vi "create_data_header_units.vi"() -> (8 "header units":string)   [LabVIEW 2016]
uses:
  Instrument_Setup.vi
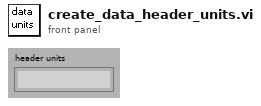
[diagram p1: front panel]
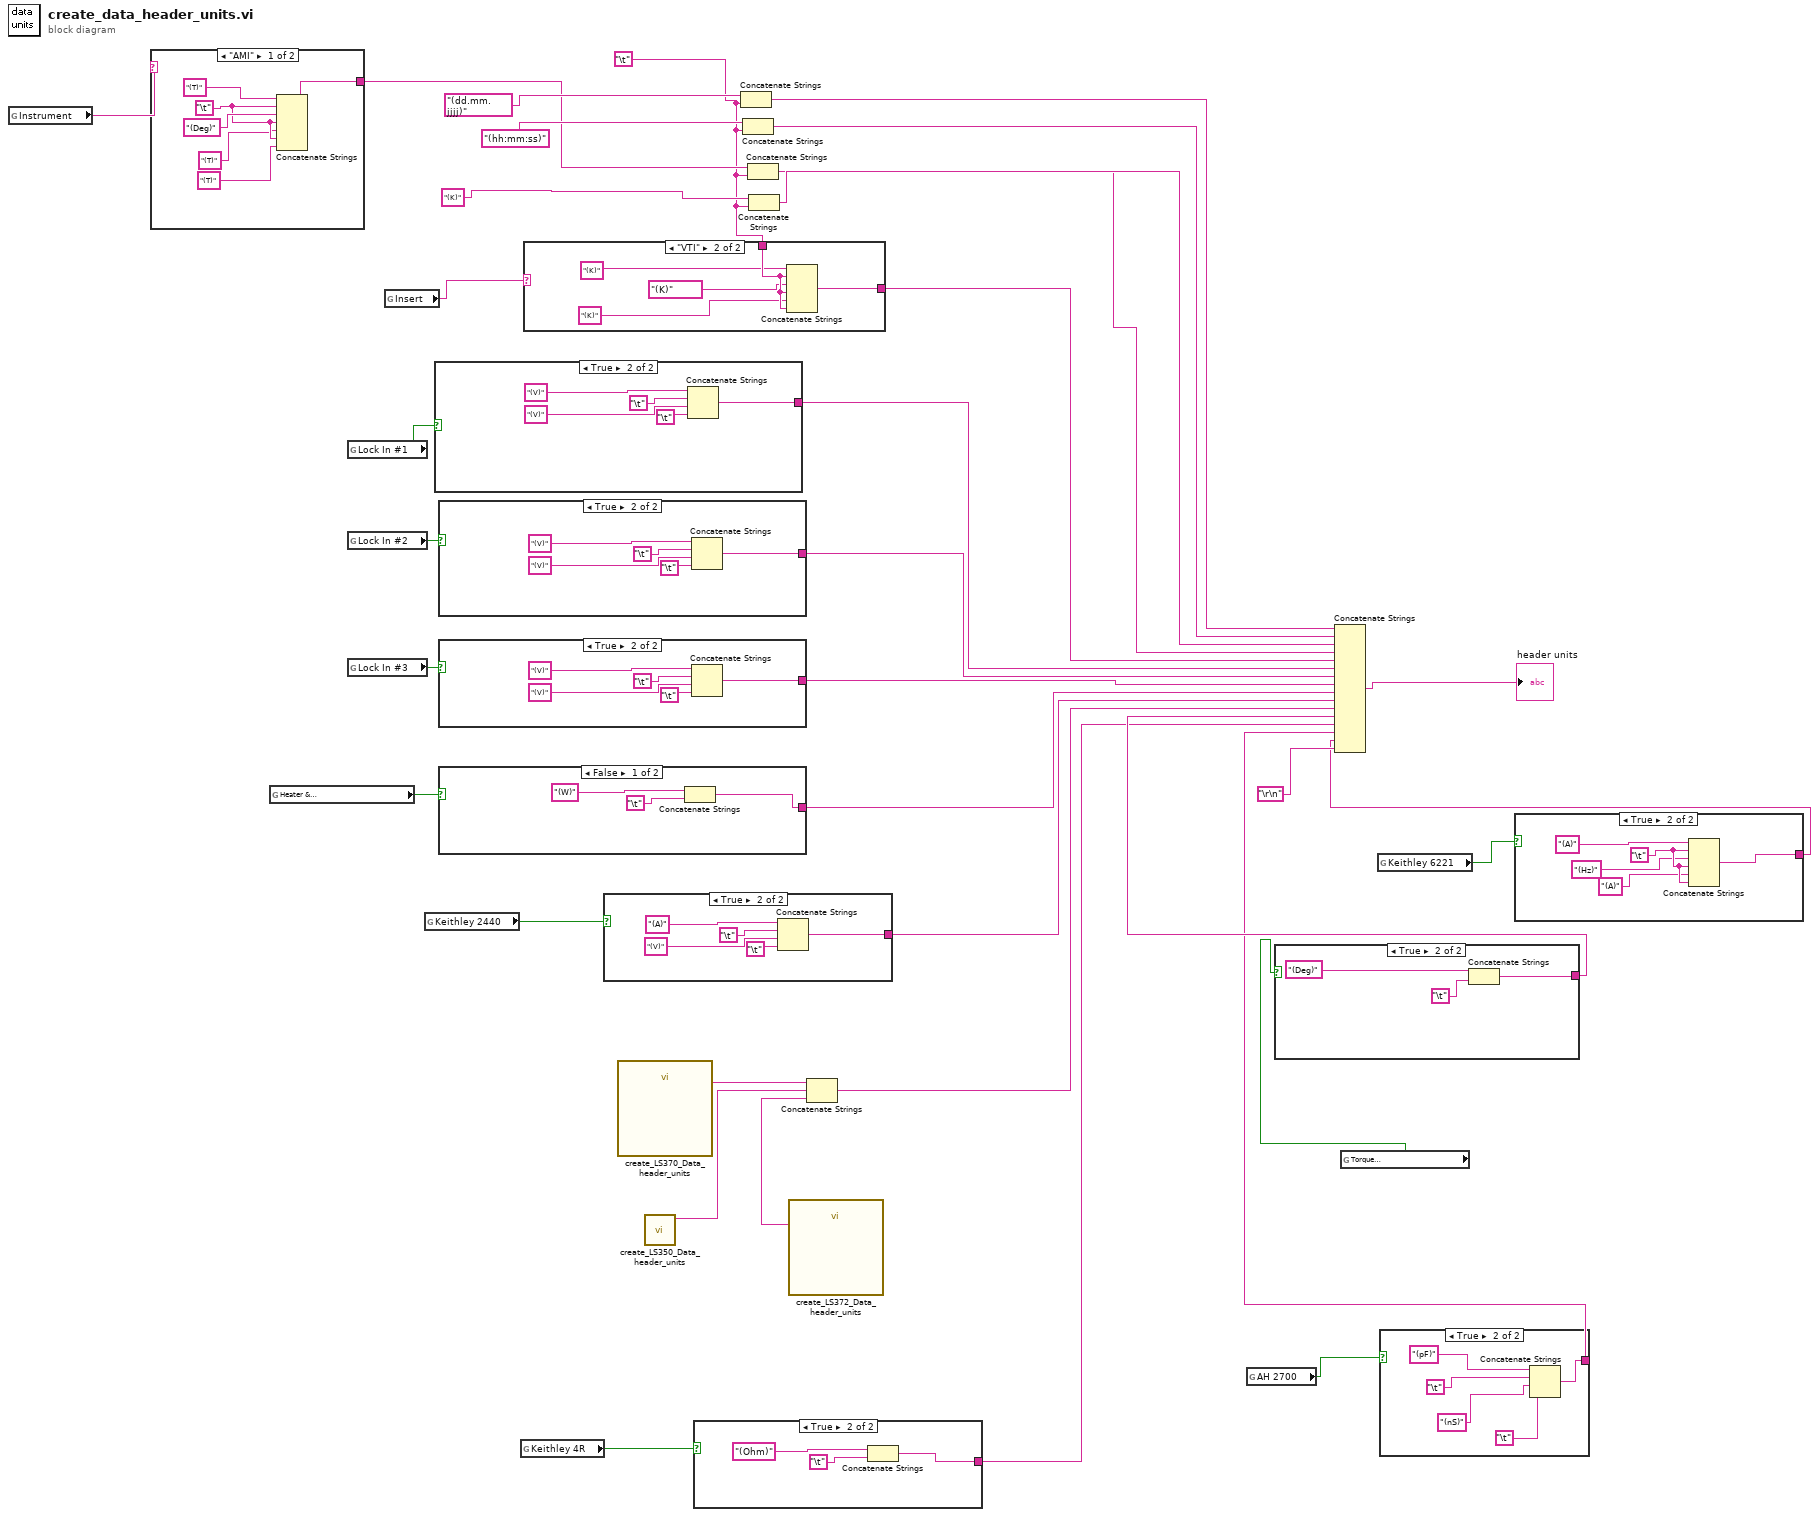
[diagram p0: block diagram]
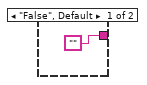
[diagram p2: hidden frame]
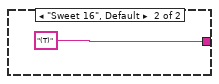
[diagram p3: hidden frame]
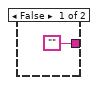
[diagram p4: hidden frame]
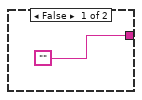
[diagram p5: hidden frame]
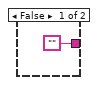
[diagram p6: hidden frame]
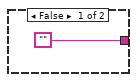
[diagram p7: hidden frame]
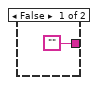
[diagram p8: hidden frame]
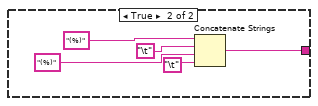
[diagram p9: hidden frame]
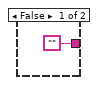
[diagram p10: hidden frame]
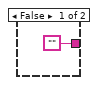
[diagram p11: hidden frame]
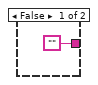
[diagram p12: hidden frame]
diagram:
  w2 = "\t"
  n1 = global read "Instrument_Setup.vi" "Instrument"() -> (w6:string)
  n2 = case shown="\"AMI\"" w6 {
    tunnel: [w40 "(T)"] -> w20
    frame "AMI" {
      w39 = "\t"
      n3 = Concatenate Strings("(T)", w39, "(Deg)", w39, "(T)", w39, "(T)") -> (w40:string)
    }
    frame "Sweet 16", Default {
    }
  }
  n4 = global read "Instrument_Setup.vi" "Heater &\nNeedle Valve"() -> (w33:bool)
  n5 = global read "Instrument_Setup.vi" "Lock In #1"() -> (w36:bool)
  n6 = global read "Instrument_Setup.vi" "Lock In #2"() -> (w35:bool)
  n7 = global read "Instrument_Setup.vi" "Lock In #3"() -> (w34:bool)
  n8 = global read "Instrument_Setup.vi" "Insert"() -> (w3:string)
  n9 = global read "Instrument_Setup.vi" "Keithley 2440"() -> (w32:bool)
  n10 = case shown="True" w36 {
    tunnel: ["" w49] -> w31
    frame False {
    }
    frame True {
      n11 = Concatenate Strings("(V)", "\t", "(V)", "\t") -> (w49:string)
    }
  }
  n12 = case shown="True" w35 {
    tunnel: ["" w51] -> w30
    frame False {
    }
    frame True {
      n13 = Concatenate Strings("(V)", "\t", "(V)", "\t") -> (w51:string)
    }
  }
  n14 = case shown="True" w34 {
    tunnel: ["" w57] -> w29
    frame False {
    }
    frame True {
      n15 = Concatenate Strings("(V)", "\t", "(V)", "\t") -> (w57:string)
    }
  }
  n16 = case shown="False" w33 {
    tunnel: [w62 w69] -> w28
    frame False {
      n17 = Concatenate Strings("(W)", "\t") -> (w62:string)
    }
    frame True {
      n18 = Concatenate Strings("(%)", "\t", "(%)", "\t") -> (w69:string)
    }
  }
  n19 = global read "Instrument_Setup.vi" "Keithley 4R"() -> (w24:bool)
  n20 = case shown="\"VTI\"" w3 {
    tunnel: w2 -> [_ w75]
    tunnel: ["" w74] -> w1
    frame "False", Default {
    }
    frame "VTI" {
      n21 = Concatenate Strings("(K)", w75, "(K)", w75, "(K)", w75) -> (w74:string)
    }
  }
  n22 = case shown="True" w32 {
    tunnel: ["" w81] -> w27
    frame False {
    }
    frame True {
      n23 = Concatenate Strings("(A)", "\t", "(V)", "\t") -> (w81:string)
    }
  }
  n24 = call "create_LS370_Data_header_units.vi"() -> ("String"=w10:string)  [unwired: 11 in]
  n25 = call "create_LS350_Data_header_units.vi"() -> ("String"=w4:string)  [unwired: 11 in]
  n26 = case shown="True" w24 {
    tunnel: ["" w85] -> w23
    frame False {
    }
    frame True {
      n27 = Concatenate Strings("(Ohm)", "\t") -> (w85:string)
    }
  }
  n28 = Concatenate Strings("(dd.mm.jjjj)", w2) -> (w17:string)
  n29 = Concatenate Strings("(hh:mm:ss)", w2) -> (w18:string)
  n30 = Concatenate Strings(w20, w2) -> (w12:string)
  n31 = Concatenate Strings("(K)", w2) -> (w13:string)
  n32 = call "create_LS372_Data_header_units.vi"() -> ("String"=w5:string)  [unwired: 11 in]
  n33 = Concatenate Strings(w10, w4, w5) -> (w9:string)
  n34 = global read "Instrument_Setup.vi" "AH 2700"() -> (w15:bool)
  n35 = global read "Instrument_Setup.vi" "Torque \nMeasurem."() -> (w25:bool)
  n36 = case shown="True" w25 {
    tunnel: ["" w89] -> w26
    frame False {
    }
    frame True {
      n37 = Concatenate Strings("(Deg)", "\t") -> (w89:string)
    }
  }
  n38 = global read "Instrument_Setup.vi" "Keithley 6221"() -> (w8:bool)
  n39 = case shown="True" w15 {
    tunnel: ["" w91] -> w14
    frame False {
    }
    frame True {
      n40 = Concatenate Strings("(pF)", "\t", "(nS)", "\t") -> (w91:string)
    }
  }
  n41 = case shown="True" w8 {
    tunnel: ["" w101] -> w7
    frame False {
    }
    frame True {
      w99 = "\t"
      n42 = Concatenate Strings("(A)", w99, "(Hz)", w99, "(A)", w99) -> (w101:string)
    }
  }
  n43 = Concatenate Strings(w17, w18, w13, w12, w1, w31, w30, w29, w28, w27, w9, w26, w23, w14, w7, "\r\n") -> (→"header units":string)
